vi "_core_repcap_channel.vi"(0 "Channel In":i32=1) -> (1 "In Range?":bool, 2 "Channel cmdValue Out":string, 3 "Channel Identifier Out":string)   [LabVIEW 2020, in "Rohde&Schwarz RTx Oscilloscopes.lvlib"]
uses:
  Rohde&Schwarz RTx Oscilloscopes.lvlib
  rsidr_core_global.vi
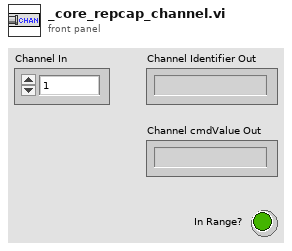
[diagram p1: front panel]
types:
  T1 = typedef "Rohde&Schwarz RTx Oscilloscopes.lvlib/rsidr_core.lvlib/type_Input_Format_RepCap.ctl" = cluster{"repCapName":string, "indetifiers":string[], "cmdValues":string[]}
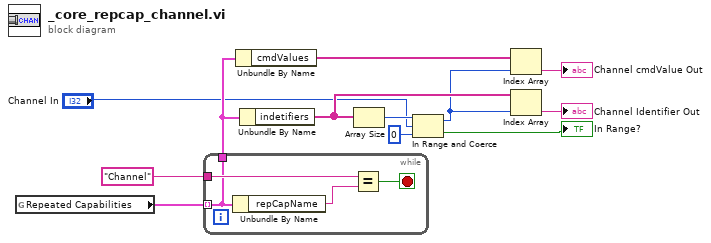
[diagram p0: block diagram]
diagram:
  n1 = global read "rsidr_core_global.vi" "Repeated Capabilities"() -> (w12:T1[])
  n2 = while {
    tunnel: w12 -> [w13] mode=indexing
    tunnel: "Channel" -> [w16]
    tunnel: [w13] -> w10
    stop <- w14 stop-if-true
    n3 = Unbundle By Name(w13) -> ("repCapName"=w15:string)
    n4 = Equal?(x=w16, y=w15) -> (x = y?=w14:bool)
  }
  n5 = Unbundle By Name(w10) -> ("cmdValues"=w7:string[])
  n6 = Unbundle By Name(w10) -> ("indetifiers"=w6:string[])
  n7 = Array Size(array=w6) -> (size(s)=w9:i32)
  n8 = In Range and Coerce(upper limit=w9, x="Channel In", lower limit=0) -> (coerced(x)=w5:i32, In Range?=→"In Range?":bool)
  n9 = Index Array(array=w7, index=w5) -> (element=→"Channel cmdValue Out":string)
  n10 = Index Array(array=w6, index=w5) -> (element=→"Channel Identifier Out":string)
